vi "LEP_RV_LaunchBuild.vi"(0 "Rebuild":bool, 11 "error in (no error)":errorcluster) -> (4 "Build Result":T1(ring), 15 "error out":errorcluster)   [LabVIEW 2011]
doc: "Loads project configuration information, creates the build folder, prepares the source files, builds, and links the embedded application."
uses:
  <vilib>/LabVIEW Targets/Embedded/ASWServer/MPU_ASWServer_Messages.ctl
  <vilib>/LabVIEW Targets/Embedded/ASWServer/MPU_ASWServer_GeneralIcons.ctl
  <vilib>/LabVIEW Targets/Embedded/ASWServer/MPU_ASWServer_GeneralCtrls.ctl
  LEP_RV_LaunchGlobals.vi
  <vilib>/LabVIEW Targets/Embedded/ASWServer/MPU_ASWServer_General_SetProgressBarValue.vi
  <vilib>/LabVIEW Targets/Embedded/ASWServer/MPU_ASWServer_General_SetProgressBarTitle.vi
panel:
  out "server build output":string
  out "Program Size":string
  out "Build Status":u32(ring)=3 items=["Build OK"=1, "Build OK, with warning(s)"=2, "Build failed with error(s)"=3, "Build cancelled"=4]
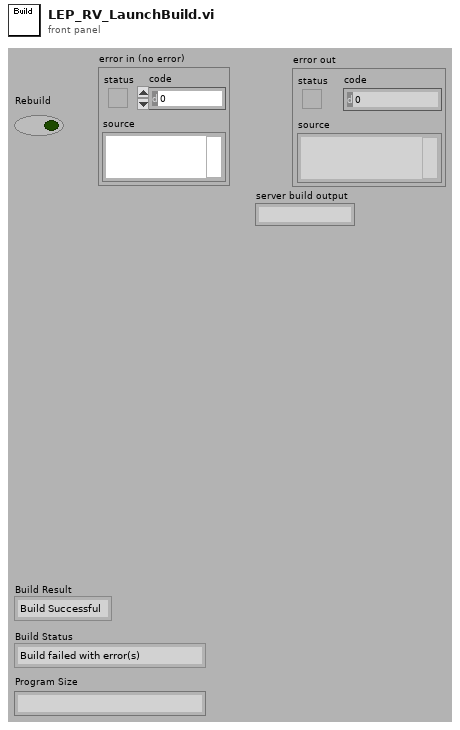
[diagram p1: front panel]
types:
  T1 = enum16{"Build Successful", "Build Failed", "Build Cancelled"}
  T2 = typedef "MPU_ASWServer_Messages.ctl" = enum32{"NoMessage", "Cancel", "ApplicationLaunched"}
  T3 = enum16{"NoErr", "TopLevelVIErr", "EmptyTopLevelVIPath", "CGenErr", "CpySuppFilesErr", "ProjectInfoErr", "NoTopLevelVIErr", "CreateBuildFolderErr", "EmptyBuildFolderErr", "LoadConfigErr", "BildToolsErr", "CompileErr", "LinkError", "DebugInfoErr", "NotFoundErr", "AccessErr", "ExecErr", "UnknownErr", "ISRErr"}
  T4 = enum16{"LoadProjectInfo", "LoadConfig", "SetupBuildFolder", "CopySupportFiles", "CGen", "CreateUVProject", "ConfigureUVproject", "BuildwithUV", "GenerateDebugDatabase", "ShowUserMessage", "Done", "Error"}
  T5 = enum32{"Unused", "OPT_LMISC", "OPT_CMISC", "OPT_AMISC", "OPT_CINCL", "OPT_AINCL", "OPT_CDEF", "OPT_ADEF", "OPT_CUNDEF", "OPT_AUNDEF", "OPT_COPTIMIZE", "OPT_CODEGEN", "OPT_MEMRANGES"}
  T6 = typedef "MPU_ASWServer_GeneralIcons.ctl" = enum16{"Complete", "Disconnected", "Error", "Initializing", "Ready", "Running", "Stopped", "Unknown", "No Change"}
  T7 = typedef "MPU_ASWServer_GeneralCtrls.ctl" = enum16{"Build Status", "Download Status", "Target Name", "Target Type", "Application Name"}
  T8 = enum32{"Unused", "OPT_LMISC", "OPT_CMISC", "OPT_AMISC", "OPT_CINCL", "OPT_AINCL", "OPT_CDEF", "OPT_ADEF", "OPT_CUNDEF", "OPT_AUNDEF", "OPT_COPTIMIZE", "OPT_CODEGEN", "OPT_MEMRANGES", "OPT_ASNMEMRANGES"}
  T9 = typedef "LEP_RV_Config.ctl" = cluster{"Enable debugging":bool, "Debug Options":u16, "Use stack variables":bool, "Generate serial only":bool, "Generate guard code":bool, "Generate Integer Only":bool, "Generate C Function Calls":bool, "ExpressionFolding":bool, "Constant Allocation":u16, "Constant Deallocation":u16, "Build Specification ID":string, "Preprocessor symbols (define)":string, "Compiler Flags":string, "Linker Flags":string, "Mode":u16, "Optimization":u16, "Optimize for time":bool, "Enable cross-module optimization":bool, "Include paths":path[], "Optimize heap size":bool, "Use MicroLib":bool, "Debug Mode":u16, "Enable profile information":bool, "Host name":string, "Use DHCP":bool, "IP address":string, "Subnet mask":string, "Gateway":string, "Primary DNS":string, "Secondary DNS":string, "MAC in target memory":bool, "MAC address":string, "Console output":u16, "Target serial port":u16}
  T10 = cluster{"region name":string, "size":u32, "max":u32, "contains heap?":bool, "RAM?":bool}[]
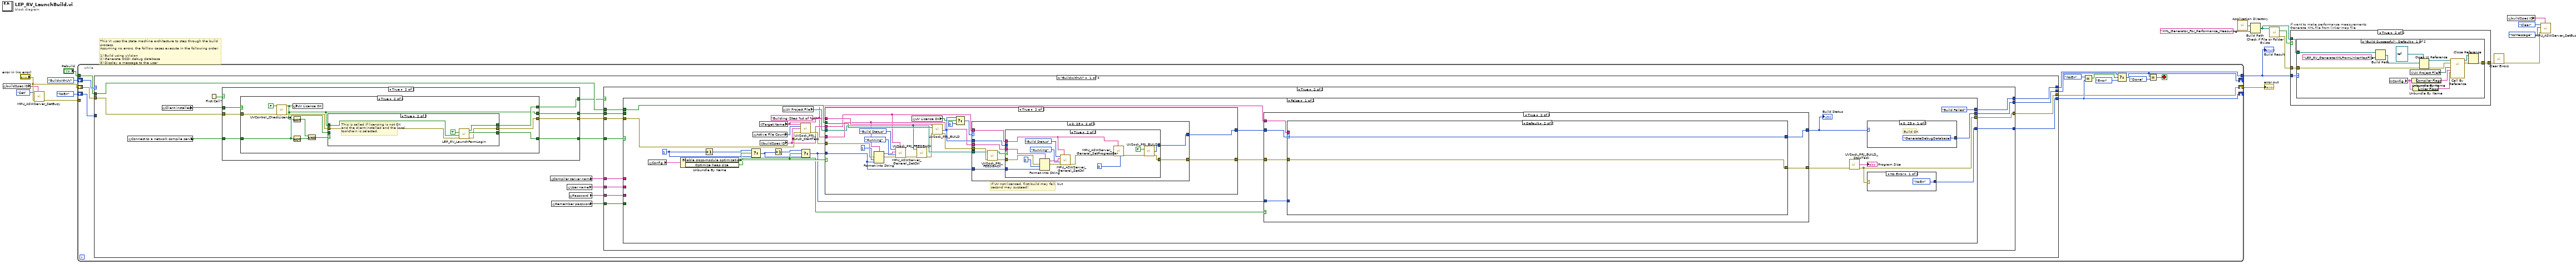
[diagram p0: block diagram]
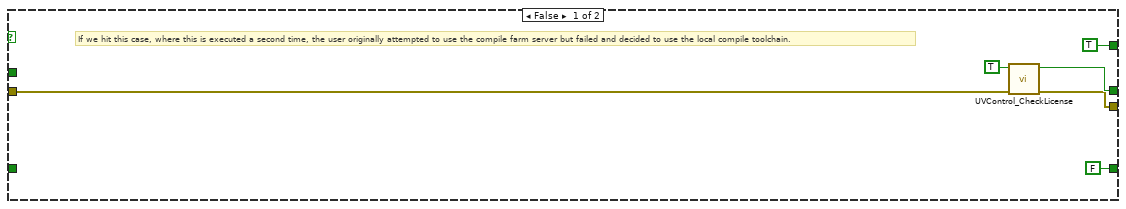
[diagram p4: hidden frame]
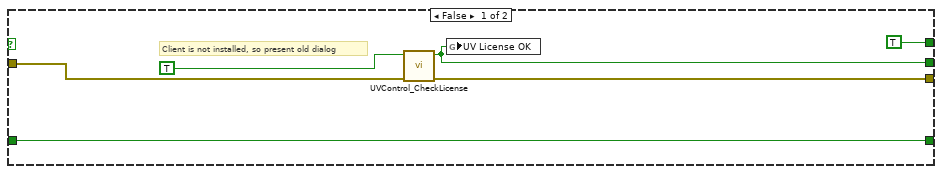
[diagram p5: hidden frame]
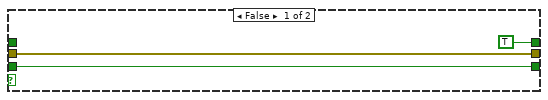
[diagram p6: hidden frame]
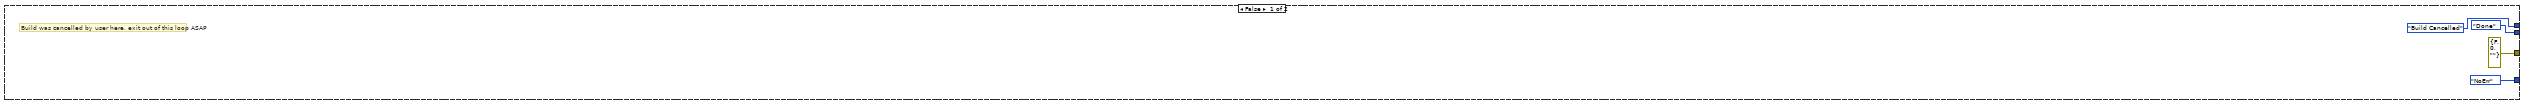
[diagram p7: hidden frame]
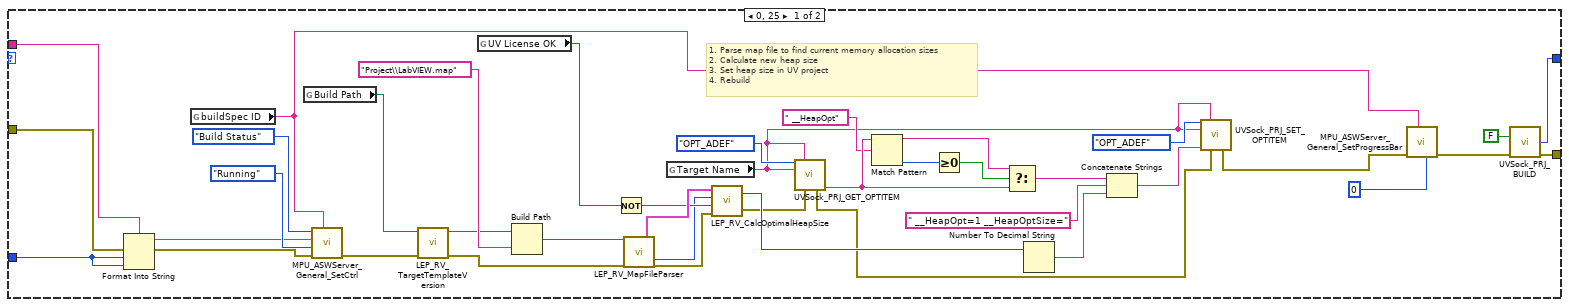
[diagram p9: hidden frame]
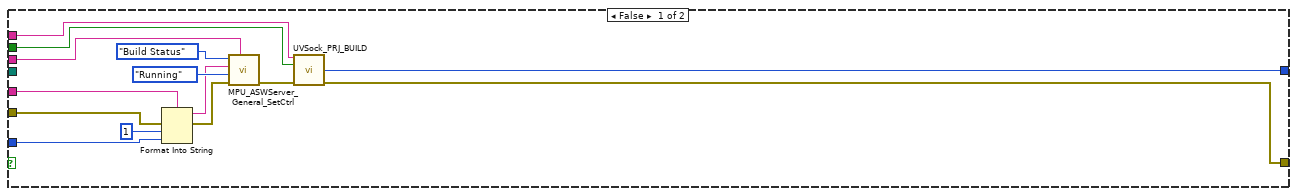
[diagram p10: hidden frame]
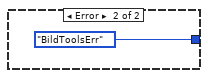
[diagram p13: hidden frame]
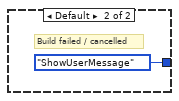
[diagram p14: hidden frame]
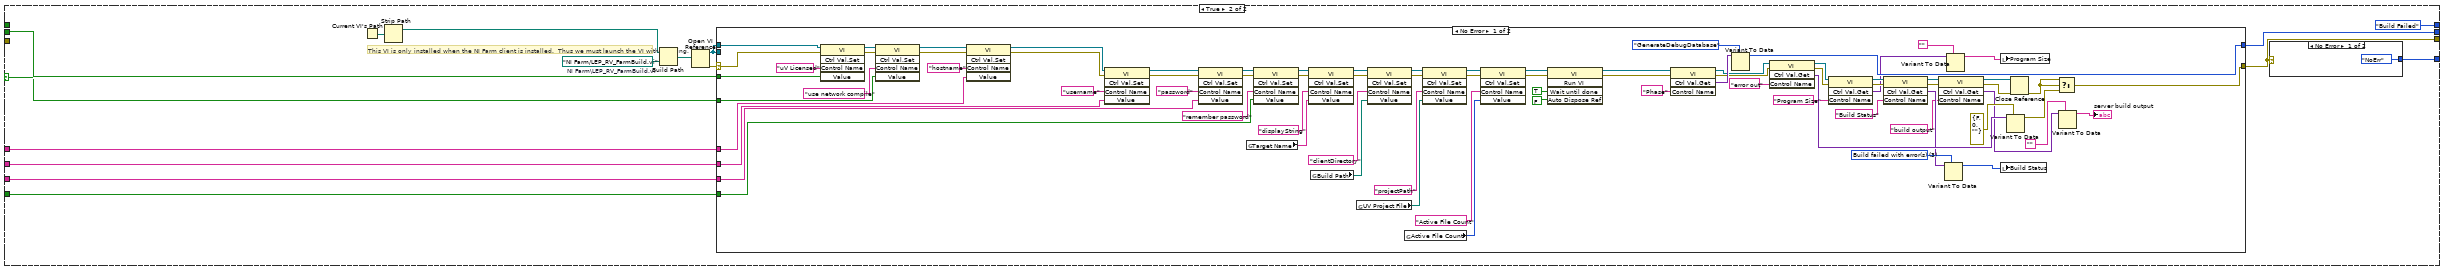
[diagram p15: hidden frame]
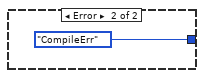
[diagram p16: hidden frame]
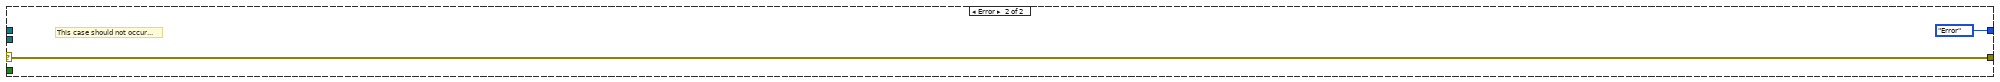
[diagram p17: hidden frame]
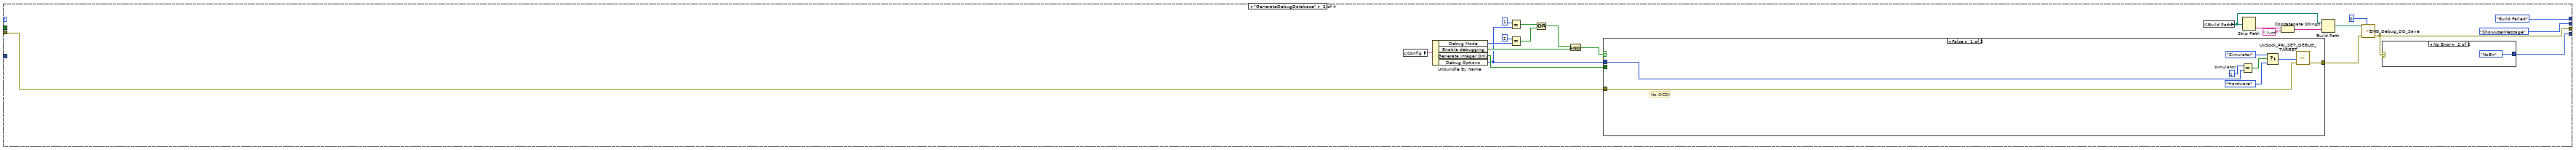
[diagram p18: hidden frame]
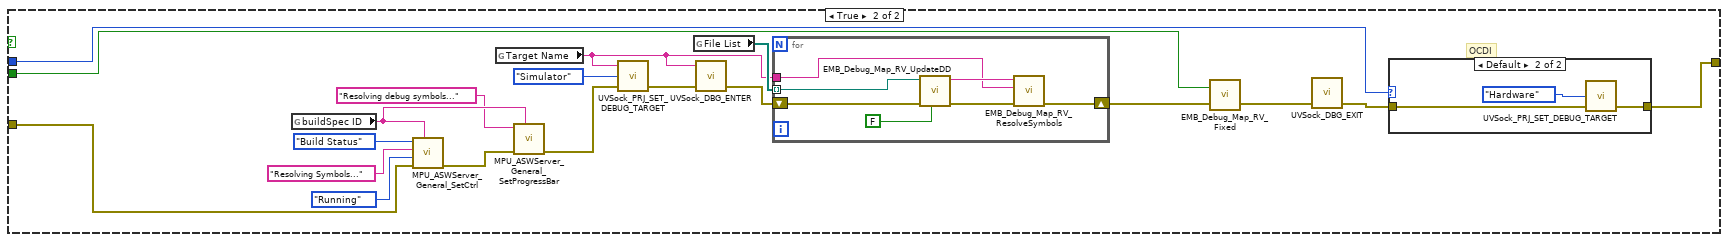
[diagram p19: hidden frame]
diagram:
  # "This VI uses the state machine architecture to step through the build process.\nAssuming no errors, the folllow cases execute in the following order:\n\n1) Build using uVision\n2) Generate OCDI debug database\n3) Display a message to the user"
  n1 = global read "LEP_RV_LaunchGlobals.vi" "buildSpec ID"() -> (w13:string)
  n2 = call <vilib>:"MPU_ASWServer_SetBusy.vi"("buildSpec ID"=w13, "error in (no error)"="error in (no error)", "action"=enum32{"Clear", "Set"}."Set") -> ("error out"=w14:errorcluster)  [unwired: 6 out]
  n3 = while {
    shift-right: [w32] -> w12
    shift-left: "error in (no error)" -> [w20]
    shift-right: [w27] -> _
    shift-left: T4."BuildwithUV" ("Phase") -> [w33]
    shift-right: [w24] -> _
    shift-left: T3."NoErr" ("Errors") -> [w31]
    tunnel: [w25] -> w2
    tunnel: "Rebuild" -> [w22]
    tunnel: w14 -> [_]
    stop <- w28 stop-if-true
    n4 = case shown="\"BuildwithUV\"" w33 {
      tunnel: w20 -> [w45 w358 w414 w539]
      tunnel: [w48 w360 w410 w539] -> w32
      tunnel: [w49 w363 w413 T3."NoErr" ("Errors")] -> w24
      tunnel: w31 -> [_ _ _ w540]
      tunnel: [w46 T4."ShowUserMessage" ("Phase") T4."Done" ("Phase") T4."Done" ("Phase")] -> w29
      tunnel: [w50 T1."Build Failed" ("Build Result") w412 T1."Build Failed" ("Build Result")] -> w25
      tunnel: w22 -> [w47 _ _ _]
      frame "BuildwithUV" {
        n5 = global read "LEP_RV_LaunchGlobals.vi" "Connect to a network compile server"() -> (w41:bool)
        n6 = global read "LEP_RV_LaunchGlobals.vi" "Client installed"() -> (w40:bool)
        n7 = First Call?() -> (First Call?: T/F=w39:bool)
        n8 = case shown="True" w39 {
          tunnel: w45 -> [w54 w63]
          tunnel: [w53 w62] -> w44
          tunnel: [FALSE ("Connect to a network compile server") w61] -> w43
          tunnel: [w55 w60] -> w42
          tunnel: [TRUE ("OK") w59] -> w34
          tunnel: w41 -> [_ w58]
          tunnel: w40 -> [_ w57]
          frame False {
            # "If we hit this case, where this is executed a second time, the user originally attempted to use the compile farm server but failed and decided to use the local compile toolchain."
            n9 = call "UVControl_CheckLicense.vi"("error in (no error)"=w54, "Show Dialog?"=TRUE) -> ("error out"=w53:errorcluster, "License OK"=w55:bool)  [unwired: 8 in]
          }
          frame True {
            n10 = case shown="True" w57 {
              tunnel: w63 -> [w69 w80]
              tunnel: [w68 w78] -> w62
              tunnel: [w65 w70] -> w60
              tunnel: w58 -> [w66 w74]
              tunnel: [w66 w76] -> w61
              tunnel: [TRUE ("OK") w73] -> w59
              frame False {
                # "Client is not installed, so present old dialog"
                n11 = call "UVControl_CheckLicense.vi"("error in (no error)"=w69, "Show Dialog?"=TRUE) -> ("error out"=w68:errorcluster, "License OK"=w65:bool)  [unwired: 8 in]
                n12 = global write "LEP_RV_LaunchGlobals.vi" "UV License OK"(w65) -> ()
              }
              frame True {
                n13 = call "UVControl_CheckLicense.vi"("error in (no error)"=w80, "Show Dialog?"=FALSE) -> ("error out"=w79:errorcluster, "License OK"=w70:bool)  [unwired: 8 in]
                n14 = Not(x=w70) -> (.not. x?=w72:bool)
                n15 = Not(x=w74) -> (.not. x?=w71:bool)
                n16 = global write "LEP_RV_LaunchGlobals.vi" "UV License OK"(w70) -> ()
                n17 = And(x=w72, y=w71) -> (x .and. y?=w75:bool)
                n18 = case shown="True" w75 {
                  tunnel: w79 -> [w83 w86]
                  tunnel: [w83 w87] -> w78
                  tunnel: w74 -> [w82 _]
                  tunnel: [w82 w88] -> w76
                  tunnel: [TRUE ("OK") w89] -> w73
                  tunnel: w70 -> [_ w84]
                  frame False {
                  }
                  frame True {
                    # "This is called if licensing is not OK\nand the client installed and the local\ntoolchain is selected."
                    n19 = call "LEP_RV_LaunchFarmLogin.vi"("error in (no error)"=w86, "uV Licensed"=w84, "build on exit"=TRUE) -> ("error out"=w87:errorcluster, "Connect to a network compile server"=w88:bool, "OK"=w89:bool)  [unwired: 5 in]
                  }
                }
              }
            }
          }
        }
        n20 = global read "LEP_RV_LaunchGlobals.vi" "Compiler server name"() -> (w38:string)
        n21 = global read "LEP_RV_LaunchGlobals.vi" "Remember password"() -> (w35:bool)
        n22 = global read "LEP_RV_LaunchGlobals.vi" "User name"() -> (w37:string)
        n23 = global read "LEP_RV_LaunchGlobals.vi" "Password"() -> (w36:string)
        n24 = case shown="True" w34 {
          tunnel: [T1."Build Cancelled" ("Build Result") w105] -> w50
          tunnel: [T3."NoErr" ("Errors") w104] -> w49
          tunnel: [errorcluster {"status"=FALSE, "code"=0, "source"=""} ("error IO") w103] -> w48
          tunnel: w47 -> [_ w102]
          tunnel: [T4."Done" ("Phase") w101] -> w46
          tunnel: w44 -> [_ w100]
          tunnel: w43 -> [_ w99]
          tunnel: w42 -> [_ w98]
          tunnel: w38 -> [_ w97]
          tunnel: w37 -> [_ w96]
          tunnel: w36 -> [_ w95]
          tunnel: w35 -> [_ w94]
          frame False {
            # "Build was cancelled by user here, exit out of this loop ASAP"
          }
          frame True {
            n25 = case shown="False" w99 {
              selector: w99 -> [_ w254]
              tunnel: [T1."Build Failed" ("Build Result") T1."Build Failed" ("Build Result")] -> w105
              tunnel: [w129 w259] -> w104
              tunnel: [w128 w257] -> w103
              tunnel: w102 -> [w127 _]
              tunnel: [w125 w256] -> w101
              tunnel: w100 -> [w106 _]
              tunnel: w98 -> [_ w255]
              tunnel: w97 -> [_ w253]
              tunnel: w96 -> [_ w252]
              tunnel: w95 -> [_ w251]
              tunnel: w94 -> [_ w250]
              frame False {
                w107 = "Building (Step %d of %d)" ("format string")
                w112 = 1
                n26 = global read "LEP_RV_LaunchGlobals.vi" "Config"() -> (w119:T9)
                n27 = Unbundle By Name(w119) -> ("Enable cross-module optimization"=w114:bool, "Optimize heap size"=w110:bool)
                n28 = Increment(x=w112) -> (x+1=w113:i32)
                n29 = Select(t=w113, s=w114, f=w112) -> (s? t:f=w109:i32)
                n30 = global read "LEP_RV_LaunchGlobals.vi" "Active File Count"() -> (w120:i32)
                n31 = global read "LEP_RV_LaunchGlobals.vi" "Target Name"() -> (w122:string)
                n32 = global read "LEP_RV_LaunchGlobals.vi" "buildSpec ID"() -> (w121:string)
                n33 = Increment(x=w109) -> (x+1=w111:i32)
                n34 = global read "LEP_RV_LaunchGlobals.vi" "UV Project File"() -> (w123:path)
                n35 = call "UVSock_PRJ_BUILD_StartTask.vi"("Target"=w122, "Active File Count"=w120, "buildSpec ID"=w121, "error in (no error)"=w106) -> ("error out"=w124:errorcluster)  [unwired: 11 out]
                n36 = Select(t=w111, s=w110, f=w109) -> (s? t:f=w108:i32)
                n37 = case shown="True" w114 {
                  tunnel: w127 -> [w193 w215]
                  tunnel: w124 -> [w183 w198]
                  tunnel: w123 -> [_ w214]
                  tunnel: [w192 w213] -> w116
                  tunnel: w122 -> [w194 w200]
                  tunnel: [w191 w212] -> w118
                  tunnel: w121 -> [w185 w195]
                  tunnel: w108 -> [w184 w196]
                  tunnel: w107 -> [w182 w197]
                  frame False {
                    n38 = Format Into String(format string=w182, error in=w183, 1, w184) -> (resulting string=w186:string, error out=w187:errorcluster)  [unwired: 1 in]
                    n39 = call <vilib>:"MPU_ASWServer_General_SetCtrl.vi"("buildSpec ID"=w185, "error in"=w187, "icon"=MPU_ASWServer_GeneralIcons."Running" ("Icon"), "value"=w186, "control"=MPU_ASWServer_GeneralCtrls."Build Status" ("Control")) -> ("error out"=w181:errorcluster)  [unwired: 4 in, 2 out]
                    n40 = call "UVSock_PRJ_BUILD.vi"("Target"=w194, "Rebuild"=w193, "error in (no error)"=w181) -> ("Build Status"=w191:u32, "error out"=w192:errorcluster)  [unwired: 11 out]
                  }
                  frame True {
                    # "If UV not licensed, first build may fail, but\nsecond may succeed!"
                    n41 = Format Into String(format string=w197, error in=w198, 1, w196) -> (resulting string=w199:string, error out=w201:errorcluster)  [unwired: 1 in]
                    n42 = call <vilib>:"MPU_ASWServer_General_SetCtrl.vi"("buildSpec ID"=w195, "error in"=w201, "icon"=MPU_ASWServer_GeneralIcons."Running" ("Icon"), "value"=w199, "control"=MPU_ASWServer_GeneralCtrls."Build Status" ("Control")) -> ("error out"=w203:errorcluster)  [unwired: 4 in, 2 out]
                    n43 = global read "LEP_RV_LaunchGlobals.vi" "UV License OK"() -> (w206:bool)
                    n44 = call "UVSock_PRJ_FEEDBACK.vi"("error in (no error)"=w203, "Path"=w214) -> ("error out"=w211:errorcluster)  [unwired: 9 out]
                    n45 = call "UVSock_PRJ_BUILD.vi"("Target"=w200, "Rebuild"=w215, "error in (no error)"=w211) -> ("Build Status"=w207:u32, "error out"=w210:errorcluster)  [unwired: 11 out]
                    n46 = Select(t=w207, s=w206, f=u32 0) -> (s? t:f=w209:u32)
                    n47 = case shown="0, 25" w209 {
                      selector: w209 -> [w217 _]
                      tunnel: w210 -> [w216 w227]
                      tunnel: w214 -> [_ w226]
                      tunnel: [w216 w224] -> w213
                      tunnel: [w217 w222] -> w212
                      tunnel: w207 -> [_ w221]
                      tunnel: w195 -> [_ w220]
                      tunnel: w197 -> [_ w219]
                      tunnel: w196 -> [_ w218]
                      frame Default {
                      }
                      frame 0, 25 {
                        n48 = call "UVSock_PRJ_FEEDBACK.vi"("error in (no error)"=w227, "Path"=w226) -> ("error out"=w225:errorcluster, "new feedback data?"=w223:bool)  [unwired: 8 out]
                        n49 = case shown="True" w223 {
                          tunnel: w225 -> [w229 w234]
                          tunnel: [w229 w244] -> w224
                          tunnel: [w228 w243] -> w222
                          tunnel: w221 -> [w228 _]
                          tunnel: w220 -> [_ w232]
                          tunnel: w219 -> [_ w231]
                          tunnel: w218 -> [_ w235]
                          frame False {
                          }
                          frame True {
                            n50 = Format Into String(format string=w231, error in=w234, 2, w235) -> (resulting string=w240:string, error out=w239:errorcluster)  [unwired: 1 in]
                            n51 = call <vilib>:"MPU_ASWServer_General_SetCtrl.vi"("buildSpec ID"=w232, "error in"=w239, "icon"=MPU_ASWServer_GeneralIcons."Running" ("Icon"), "value"=w240, "control"=MPU_ASWServer_GeneralCtrls."Build Status" ("Control")) -> ("error out"=w233:errorcluster)  [unwired: 4 in, 2 out]
                            n52 = call-poly <vilib>:"MPU_ASWServer_General_SetProgressBar.vi"("value"=u32 0, "buildSpec ID"=w232, "error in"=w233) -> ("error out"=w242:errorcluster)  [unwired: 6 in, 2 out]
                            n53 = call "UVSock_PRJ_BUILD.vi"("Rebuild"=FALSE, "error in (no error)"=w242) -> ("Build Status"=w243:u32, "error out"=w244:errorcluster)  [unwired: 1 in, 11 out]
                          }
                        }
                      }
                    }
                  }
                }
                n54 = case shown="True" w110 {
                  tunnel: w118 -> [w132 w138]
                  tunnel: w116 -> [w131 w136]
                  tunnel: [w132 w137] -> w117
                  tunnel: [w131 w135] -> w115
                  tunnel: w108 -> [_ w134]
                  tunnel: w107 -> [_ w133]
                  frame False {
                  }
                  frame True {
                    n55 = case shown="Default" w138 {
                      selector: w138 -> [_ w180]
                      tunnel: [w172 w180] -> w137
                      tunnel: w136 -> [w153 w179]
                      tunnel: [w173 w179] -> w135
                      tunnel: w134 -> [w152 _]
                      tunnel: w133 -> [w151 _]
                      frame 0, 25 {
                        # "1. Parse map file to find current memory allocation sizes\n2. Calculate new heap size\n3. Set heap size in UV project\n4. Rebuild"
                        n56 = Format Into String(format string=w151, error in=w153, w152, w152) -> (resulting string=w156:string, error out=w157:errorcluster)  [unwired: 1 in]
                        n57 = global read "LEP_RV_LaunchGlobals.vi" "buildSpec ID"() -> (w155:string)
                        n58 = global read "LEP_RV_LaunchGlobals.vi" "Build Path"() -> (w178:path)
                        n59 = call <vilib>:"MPU_ASWServer_General_SetCtrl.vi"("buildSpec ID"=w155, "error in"=w157, "icon"=MPU_ASWServer_GeneralIcons."Running" ("Icon"), "value"=w156, "control"=MPU_ASWServer_GeneralCtrls."Build Status" ("Control")) -> ("error out"=w154:errorcluster)  [unwired: 4 in, 2 out]
                        n60 = call "LEP_RV_TargetTemplateVersion.vi"("error in (no error)"=w154, "Path"=w178) -> ("error out"=w175:errorcluster, "Path plus Version"=w176:path)  [unwired: 7 in, 1 out]
                        n61 = global read "LEP_RV_LaunchGlobals.vi" "UV License OK"() -> (w162:bool)
                        n62 = Build Path(base path=w176, name or relative path="Project\\LabVIEW.map") -> (appended path=w174:path)
                        n63 = Not(x=w162) -> (.not. x?=w161:bool)
                        n64 = call "LEP_RV_MapFileParser.vi"("map file"=w174, "error in (no error)"=w175) -> ("regions"=w164:T10, "heap size"=w160:i32, "error out"=w163:errorcluster)  [unwired: 11 in, 4 out]
                        n65 = global read "LEP_RV_LaunchGlobals.vi" "Target Name"() -> (w141:string)
                        n66 = call "LEP_RV_CalcOptimalHeapSize.vi"("error in (no error)"=w163, "eval mode?"=w161, "heap size"=w160, "memory regions"=w164) -> ("error out"=w140:errorcluster, "optimal heap size"=w165:u32)
                        n67 = call "UVSock_PRJ_GET_OPTITEM.vi"("Option In"=T5."OPT_ADEF", "Target"=w141, "Target Name In"=w141, "error in (no error)"=w140) -> ("error out"=w139:errorcluster, "Item Out"=w148:string)  [unwired: 9 in, 1 out]
                        n68 = Match Pattern(string=w148, regular expression=" __HeapOpt") -> (before substring=w149:string, offset past match=w147:i32)  [unwired: 1 in, 2 out]
                        n69 = Greater Or Equal To 0?(x=w147) -> (x >= 0?=w146:bool)
                        n70 = Select(t=w149, s=w146, f=w148) -> (s? t:f=w143:string)
                        n71 = Number To Decimal String(number=w165) -> (decimal integer string=w167:string)  [unwired: 1 in]
                        n72 = Concatenate Strings(w143, " __HeapOpt=1 __HeapOptSize=" ("string"), w167) -> (w142:string)
                        n73 = call "UVSock_PRJ_SET_OPTITEM.vi"("Option In"=T8."OPT_ADEF", "Target"=w141, "Target Name In"=w141, "Item In"=w142, "error in (no error)"=w139) -> ("error out"=w168:errorcluster)  [unwired: 10 in]
                        n74 = call-poly <vilib>:"MPU_ASWServer_General_SetProgressBar.vi"("value"=u32 0, "buildSpec ID"=w155, "error in"=w168) -> ("error out"=w170:errorcluster)  [unwired: 6 in, 2 out]
                        n75 = call "UVSock_PRJ_BUILD.vi"("Rebuild"=FALSE, "error in (no error)"=w170) -> ("Build Status"=w172:u32, "error out"=w173:errorcluster)  [unwired: 1 in, 11 out]
                      }
                      frame Default {
                      }
                    }
                  }
                }
                "Build Status" <- w117
                n76 = call "UVSock_PRJ_BUILD_StopTask.vi"("error in (no error)"=w115) -> ("error out"=w128:errorcluster, "Program Size"=→"Program Size":string)  [unwired: 3 out]
                n77 = case shown="0, 25" w117 {
                  tunnel: [T4."GenerateDebugDatabase" ("Phase") T4."ShowUserMessage" ("Phase")] -> w125
                  frame 0, 25 {
                    # "Build OK"
                  }
                  frame Default {
                    # "Build failed / cancelled"
                  }
                }
                n78 = case shown="No Error" w128 {
                  tunnel: [T3."NoErr" ("Errors") T3."BildToolsErr" ("Errors")] -> w129
                  frame No Error {
                  }
                  frame Error {
                  }
                }
              }
              frame True {
                w264 = path "NI Farm/LEP_RV_FarmBuild.vi"  # NI Farm\LEP_RV_FarmBuild.vi
                # "This VI is only installed when the NI Farm client is installed.  Thus we must launch the VI with scripting."
                n79 = Current VI's Path() -> (path=w263:path)
                n80 = Strip Path(path=w263) -> (stripped path=w262:path)  [unwired: 1 out]
                n81 = Build Path(base path=w262, name or relative path=w264) -> (appended path=w261:path)
                n82 = Open VI Reference(vi path=w261) -> (vi reference=w249:refnum<vi>, error out=w260:errorcluster)  [unwired: 5 in]
                n83 = case shown="No Error" w260 {
                  selector: w260 -> [w338 w346]
                  tunnel: w249 -> [w339 _]
                  tunnel: [w325 w346] -> w257
                  tunnel: [w333 T4."Error" ("Phase")] -> w256
                  tunnel: w255 -> [w337 _]
                  tunnel: w254 -> [w303 _]
                  tunnel: w253 -> [w302 _]
                  tunnel: w252 -> [w301 _]
                  tunnel: w251 -> [w300 _]
                  tunnel: w250 -> [w299 _]
                  tunnel: w249 -> [_ _]
                  frame No Error {
                    w283 = u32 3 items=["Build OK"=1, "Build OK, with warning(s)"=2, "Build failed with error(s)"=3, "Build cancelled"=4] ("Build Status")
                    n84 = invoke class="VI" method="Ctrl Val.Set"(reference=w339, error in=w338, "Control Name"="uV Licensed", "Value"=w337) -> (reference out=w305:refnum<vi>, error out=w304:errorcluster)  [unwired: 1 in, 3 out]
                    n85 = invoke class="VI" method="Ctrl Val.Set"(reference=w305, error in=w304, "Control Name"="use network compile", "Value"=w303) -> (reference out=w309:refnum<vi>, error out=w308:errorcluster)  [unwired: 1 in, 3 out]
                    n86 = invoke class="VI" method="Ctrl Val.Set"(reference=w309, error in=w308, "Control Name"="hostname", "Value"=w302) -> (reference out=w311:refnum<vi>, error out=w310:errorcluster)  [unwired: 1 in, 3 out]
                    n87 = invoke class="VI" method="Ctrl Val.Set"(reference=w311, error in=w310, "Control Name"="username", "Value"=w301) -> (reference out=w313:refnum<vi>, error out=w312:errorcluster)  [unwired: 1 in, 3 out]
                    n88 = invoke class="VI" method="Ctrl Val.Set"(reference=w313, error in=w312, "Control Name"="password", "Value"=w300) -> (reference out=w315:refnum<vi>, error out=w314:errorcluster)  [unwired: 1 in, 3 out]
                    n89 = global read "LEP_RV_LaunchGlobals.vi" "Target Name"() -> (w297:string)
                    n90 = invoke class="VI" method="Ctrl Val.Set"(reference=w315, error in=w314, "Control Name"="remember password", "Value"=w299) -> (reference out=w317:refnum<vi>, error out=w316:errorcluster)  [unwired: 1 in, 3 out]
                    n91 = invoke class="VI" method="Ctrl Val.Set"(reference=w317, error in=w316, "Control Name"="displayString", "Value"=w297) -> (reference out=w307:refnum<vi>, error out=w306:errorcluster)  [unwired: 1 in, 3 out]
                    n92 = global read "LEP_RV_LaunchGlobals.vi" "Build Path"() -> (w298:path)
                    n93 = global read "LEP_RV_LaunchGlobals.vi" "UV Project File"() -> (w293:path)
                    n94 = invoke class="VI" method="Ctrl Val.Set"(reference=w307, error in=w306, "Control Name"="clientDirectory", "Value"=w298) -> (reference out=w296:refnum<vi>, error out=w295:errorcluster)  [unwired: 1 in, 3 out]
                    n95 = global read "LEP_RV_LaunchGlobals.vi" "Active File Count"() -> (w275:i32)
                    n96 = invoke class="VI" method="Ctrl Val.Set"(reference=w296, error in=w295, "Control Name"="projectPath", "Value"=w293) -> (reference out=w280:refnum<vi>, error out=w279:errorcluster)  [unwired: 1 in, 3 out]
                    n97 = invoke class="VI" method="Ctrl Val.Set"(reference=w280, error in=w279, "Control Name"="Active File Count", "Value"=w275) -> (reference out=w278:refnum<vi>, error out=w277:errorcluster)  [unwired: 1 in, 3 out]
                    n98 = invoke class="VI" method="Run VI"(reference=w278, error in=w277, "Wait until done"=TRUE ("Wait Until Done"), "Auto Dispose Ref"=FALSE ("Auto Dispose Reference")) -> (reference out=w342:refnum<vi>, error out=w341:errorcluster)  [unwired: 1 in, 3 out]
                    n99 = invoke class="VI" method="Ctrl Val.Get"(reference=w342, error in=w341, "Control Name"="Phase") -> (reference out=w332:refnum<vi>, error out=w331:errorcluster, "Get Control Value Variant"=w334:variant)  [unwired: 1 in, 1 out]
                    n100 = Variant To Data(type=T4."GenerateDebugDatabase" ("Phase"), Variant=w334) -> (data=w333:T4)  [unwired: 1 in, 1 out]
                    n101 = invoke class="VI" method="Ctrl Val.Get"(reference=w332, error in=w331, "Control Name"="error out") -> (reference out=w292:refnum<vi>, error out=w290:errorcluster, "Get Control Value Variant"=w328:variant)  [unwired: 1 in, 1 out]
                    n102 = invoke class="VI" method="Ctrl Val.Get"(reference=w292, error in=w290, "Control Name"="Program Size") -> (reference out=w291:refnum<vi>, error out=w289:errorcluster, "Get Control Value Variant"=w285:variant)  [unwired: 1 in, 1 out]
                    n103 = invoke class="VI" method="Ctrl Val.Get"(reference=w291, error in=w289, "Control Name"="Build Status") -> (reference out=w274:refnum<vi>, error out=w273:errorcluster, "Get Control Value Variant"=w282:variant)  [unwired: 1 in, 1 out]
                    n104 = invoke class="VI" method="Ctrl Val.Get"(reference=w274, error in=w273, "Control Name"="build output") -> (reference out=w272:refnum<vi>, error out=w271:errorcluster, "Get Control Value Variant"=w269:variant)  [unwired: 1 in, 1 out]
                    n105 = Variant To Data(type=w283, Variant=w282) -> (data=w281:u32)  [unwired: 1 in, 1 out]
                    n106 = Variant To Data(type="" ("Program Size"), Variant=w285) -> (data=w284:string)  [unwired: 1 in, 1 out]
                    n107 = local write "Program Size"(w284) -> ()
                    n108 = local write "Build Status"(w281) -> ()
                    n109 = Variant To Data(type=errorcluster {"status"=FALSE, "code"=0, "source"=""} ("error out"), Variant=w328) -> (data=w326:errorcluster)  [unwired: 1 in, 1 out]
                    n110 = Close Reference(reference=w272, error in (no error)=w271) -> (error out=w327:errorcluster)
                    n111 = Select(t=w327, s=w327, f=w326) -> (s? t:f=w325:errorcluster)
                    n112 = Variant To Data(type="", Variant=w269) -> (data=→"server build output":string)  [unwired: 1 in, 1 out]
                  }
                  frame Error {
                    # "This case should not occur..."
                  }
                }
                n113 = case shown="No Error" w257 {
                  tunnel: [T3."NoErr" ("Errors") T3."CompileErr" ("Errors")] -> w259
                  frame No Error {
                  }
                  frame Error {
                  }
                }
              }
            }
          }
        }
      }
      frame "GenerateDebugDatabase" {
        n114 = global read "LEP_RV_LaunchGlobals.vi" "Config"() -> (w348:T9)
        n115 = Unbundle By Name(w348) -> ("Debug Mode"=w354:u16, "Enable debugging"=w356:bool, "Generate Integer Only"=w359:bool, "Debug Options"=w349:u16)
        n116 = Equal?(x=u16 1, y=w349) -> (x = y?=w351:bool)
        n117 = Equal?(x=u16 2, y=w354) -> (x = y?=w355:bool)
        n118 = Or(x=w351, y=w355) -> (x .or. y?=w352:bool)
        n119 = And(x=w352, y=w356) -> (x .and. y?=w357:bool)
        n120 = case shown="False" w357 {
          tunnel: w358 -> [w377 w386]
          tunnel: [w376 w385] -> w361
          tunnel: w359 -> [_ w395]
          tunnel: w349 -> [w371 w391]
          frame False {
            w370 = u16 1  # simulator
            # "No OCDI"
            n121 = Equal?(x=w370, y=w371) -> (x = y?=w372:bool)
            n122 = Select(t=enum16{"Hardware", "Simulator"}."Simulator" ("Debug Target"), s=w372, f=enum16{"Hardware", "Simulator"}."Hardware") -> (s? t:f=w374:enum16{"Hardware", "Simulator"})
            n123 = call "UVSock_PRJ_SET_DEBUG_TARGET.vi"("error in (no error)"=w377, "Debug Target"=w374) -> ("error out"=w376:errorcluster)  [unwired: 1 in, 2 out]
          }
          frame True {
            # "OCDI"
            n124 = global read "LEP_RV_LaunchGlobals.vi" "buildSpec ID"() -> (w379:string)
            n125 = call <vilib>:"MPU_ASWServer_General_SetCtrl.vi"("buildSpec ID"=w379, "error in"=w386, "icon"=MPU_ASWServer_GeneralIcons."Running" ("Icon"), "value"="Resolving Symbols...", "control"=MPU_ASWServer_GeneralCtrls."Build Status" ("Control")) -> ("error out"=w381:errorcluster)  [unwired: 4 in, 2 out]
            n126 = global read "LEP_RV_LaunchGlobals.vi" "Target Name"() -> (w382:string)
            n127 = call-poly <vilib>:"MPU_ASWServer_General_SetProgressBar.vi"("buildSpec ID"=w379, "error in"=w381, "title"="Resolving debug symbols...") -> ("error out"=w380:errorcluster)  [unwired: 6 in, 2 out]
            n128 = call "UVSock_PRJ_SET_DEBUG_TARGET.vi"("error in (no error)"=w380, "Debug Target"=enum16{"Hardware", "Simulator"}."Simulator", "Target"=w382) -> ("error out"=w393:errorcluster)  [unwired: 2 out]
            n129 = global read "LEP_RV_LaunchGlobals.vi" "File List"() -> (w383:path[])
            n130 = call "UVSock_DBG_ENTER.vi"("error in (no error)"=w393, "Target"=w382) -> ("error out"=w384:errorcluster)  [unwired: 3 out]
            n131 = for {
              tunnel: w383 -> [w404] mode=indexing
              shift-right: [w402] -> w396
              shift-left: w384 -> [w407]
              tunnel: w382 -> [w401]
              n132 = call "EMB_Debug_Map_RV_UpdateDD.vi"("RDM"=FALSE, "error in (no error)"=w407, "Source Path"=w404) -> ("error out"=w405:errorcluster, "VI Name"=w403:string)  [unwired: 2 in, 5 out]
              n133 = call "EMB_Debug_Map_RV_ResolveSymbols.vi"("error in (no error)"=w405, "Target"=w401, "VI Name"=w403) -> ("error out"=w402:errorcluster)  [unwired: 8 out]
            }
            n134 = call "EMB_Debug_Map_RV_Fixed.vi"("error in (no error)"=w396, "Generate Integer Only"=w395) -> ("error out"=w394:errorcluster)  [unwired: 1 out]
            n135 = call "UVSock_DBG_EXIT.vi"("error in (no error)"=w394) -> ("error out"=w390:errorcluster)  [unwired: 1 in, 3 out]
            n136 = case shown="Default" w391 {
              tunnel: w390 -> [w397 w399]
              tunnel: [w397 w398] -> w385
              frame 1 {
              }
              frame Default {
                n137 = call "UVSock_PRJ_SET_DEBUG_TARGET.vi"("error in (no error)"=w399, "Debug Target"=enum16{"Hardware", "Simulator"}."Hardware") -> ("error out"=w398:errorcluster)  [unwired: 1 in, 2 out]
              }
            }
          }
        }
        n138 = global read "LEP_RV_LaunchGlobals.vi" "Build Path"() -> (w347:path)
        n139 = Strip Path(path=w347) -> (name=w366:string)  [unwired: 1 out]
        n140 = Concatenate Strings(w366, ".lvm" ("name or relative path")) -> (w368:string)
        n141 = Build Path(base path=w347, name or relative path=w368) -> (appended path=w365:path)
        n142 = call <vilib>:"EMB_Debug_DD_Save.vi"("target ID"=u32 0, "error in (no error)"=w361, "Path"=w365) -> ("error out"=w360:errorcluster)  [unwired: 8 out]
        n143 = case shown="No Error" w360 {
          tunnel: [T3."NoErr" ("Errors") T3."DebugInfoErr" ("Errors")] -> w363
          frame No Error {
          }
          frame Error {
          }
        }
      }
      frame "ShowUserMessage" {
        n144 = case "Show the correct dialogs for the build result" shown="No Error" w414 {
          tunnel: [T3."NoErr" ("Errors") T3."BildToolsErr" ("Errors")] -> w413
          tunnel: [w422 T1."Build Failed" ("Build Result")] -> w412
          tunnel: [w418 _] -> w410
          frame No Error {
            n145 = global read "LEP_RV_LaunchGlobals.vi" "buildSpec ID"() -> (w415:string)
            n146 = local read "Program Size"() -> (w420:string)
            n147 = local read "Build Status"() -> (w421:u32)
            n148 = call-poly <vilib>:"MPU_ASWServer_General_SetProgressBar.vi"("value"=u32 0, "buildSpec ID"=w415) -> ("error out"=w417:errorcluster)  [unwired: 7 in, 2 out]
            n149 = case shown="26, Default" w421 {
              tunnel: [T1."Build Successful" ("Build Result") T1."Build Failed" ("Build Result") T1."Build Cancelled" ("Build Result")] -> w422
              tunnel: w420 -> [_ _ _]
              tunnel: w415 -> [w426 w461 w500]
              tunnel: [w439 errorcluster {"status"=TRUE, "code"=42, "source"="failed"} ("error out") errorcluster {"status"=TRUE, "code"=42, "source"="Cancelled"} ("error out")] -> w418
              tunnel: w417 -> [w442 w484 w507]
              frame 0, 25 {
                w427 = "Build Report" ("tab name")
                w449 = "Output" ("tab name")
                n150 = Get Date/Time In Seconds() -> (seconds since 1Jan1904=w444:timestamp)
                n151 = Get Date/Time String(seconds (now)=w444, want seconds? (F)=TRUE) -> (time string=w448:string)  [unwired: 2 out]
                n152 = Concatenate Strings("[" ("string"), w448, "]" ("string"), " Status: Build Succeeded." ("string"), "\r\n") -> (w452:string)
                n153 = call <vilib>:"MPU_ASWServer_Send.vi"("generate events? (F)"=TRUE ("show tab? (F)"), "wait for ACK (T)"=FALSE, "buildSpec ID"=w426, "error in"=w442, "control value"=w452, "control name"=w449, "tab name"=w449) -> ("error out"=w441:errorcluster)  [unwired: 4 out]
                n154 = global read "LEP_RV_LaunchGlobals.vi" "UV License OK"() -> (w429:bool)
                n155 = call-poly <vilib>:"MPU_ASWServer_General_SetProgressBar.vi"("buildSpec ID"=w426, "error in"=w441, "title"="Done") -> ("error out"=w453:errorcluster)  [unwired: 6 in, 2 out]
                n156 = call <vilib>:"MPU_ASWServer_General_SetCtrl.vi"("buildSpec ID"=w426, "error in"=w453, "icon"=MPU_ASWServer_GeneralIcons."Running" ("Icon"), "value"="Build Succeeded" ("Value"), "control"=MPU_ASWServer_GeneralCtrls."Build Status" ("Control")) -> ("error out"=w431:errorcluster)  [unwired: 4 in, 2 out]
                n157 = Not(x=w429) -> (.not. x?=w428:bool)
                n158 = global read "LEP_RV_LaunchGlobals.vi" "Build Path"() -> (w433:path)
                n159 = call "LEP_RV_TargetTemplateVersion.vi"("Path"=w433) -> ("Path plus Version"=w432:path)  [unwired: 8 in, 2 out]
                n160 = call <vilib>:"MPU_ASWServer_Send.vi"("generate events? (F)"=FALSE, "wait for ACK (T)"=FALSE, "buildSpec ID"=w426, "error in"=w431, "control value"=w428, "control name"="eval mode?", "tab name"=w427) -> ("error out"=w430:errorcluster)  [unwired: 4 out]
                n161 = Build Path(base path=w432, name or relative path="Project\\LabVIEW.map") -> (appended path=w434:path)
                n162 = call <vilib>:"MPU_ASWServer_Send.vi"("generate events? (F)"=TRUE, "wait for ACK (T)"=FALSE, "buildSpec ID"=w426, "error in"=w430, "control value"=w434, "control name"="path to map file", "tab name"=w427) -> ("error out"=w439:errorcluster)  [unwired: 4 out]
              }
              frame 26, Default {
                w482 = "\r\n"
                n163 = global read "LEP_RV_LaunchGlobals.vi" "Connect to a network compile server"() -> (w459:bool)
                n164 = case shown="False" w459 {
                  tunnel: [w493 w494] -> w478
                  frame False {
                    n165 = call "UVSock_GetBuildOutput.vi"() -> ("Build Output"=w493:string)  [unwired: 2 in, 3 out]
                  }
                  frame True {
                    n166 = local read "server build output"() -> (w494:string)
                  }
                }
                n167 = Match Pattern(string=w478, regular expression="linking...") -> (before substring=w473:string, match substring=w475:string, after substring=w474:string, offset past match=w476:i32)  [unwired: 1 in]
                n168 = case shown="Default" w476 {
                  tunnel: w475 -> [w497 _]
                  tunnel: w474 -> [w496 _]
                  tunnel: w473 -> [_ w498]
                  tunnel: [w495 w498] -> w469
                  frame Default {
                    n169 = Concatenate Strings(w497, w496) -> (w495:string)
                  }
                  frame -1 {
                  }
                }
                n170 = Match Pattern(string=w469, regular expression="L6406W") -> (offset past match=w471:i32)  [unwired: 1 in, 3 out]
                n171 = Greater Or Equal To 0?(x=w471) -> (x >= 0?=w470:bool)
                n172 = Select(t="linking...\nError: Application is too large for target memory.", s=w470, f=w469) -> (s? t:f=w467:string)
                n173 = Concatenate Strings(w467, w482, "Status: Build failed." ("string"), w482) -> (w481:string)
                n174 = call <vilib>:"MPU_ASWServer_General_SetCtrl.vi"("buildSpec ID"=w461, "error in"=w484, "icon"=MPU_ASWServer_GeneralIcons."Error", "value"="Build Failed", "control"=MPU_ASWServer_GeneralCtrls."Build Status") -> ("error out"=w488:errorcluster)  [unwired: 4 in, 2 out]
                n175 = String Subset(string=w481, length (rest)=30000 ("length (rest)")) -> (substring=w480:string)  [unwired: 1 in]
                n176 = call-poly <vilib>:"MPU_ASWServer_General_SetProgressBar.vi"("buildSpec ID"=w461, "error in"=w488, "title"="Failed") -> ("error out"=w489:errorcluster)  [unwired: 6 in, 2 out]
                n177 = call <vilib>:"MPU_ASWServer_Output_SetError.vi"("error in"=w489, "error str"=w480, "buildSpec ID"=w461) -> ("error out"=w462:errorcluster)  [unwired: 2 in, 4 out]
                n178 = call <vilib>:"MPU_ASWServer_Send.vi"("generate events? (F)"=TRUE, "wait for ACK (T)"=FALSE, "buildSpec ID"=w461, "error in"=w462, "control value"=path "", "control name"="path to map file", "tab name"="Build Report") -> ()  [unwired: 5 out]
              }
              frame 27 {
                w515 = "Output" ("tab name")
                n179 = Get Date/Time In Seconds() -> (seconds since 1Jan1904=w509:timestamp)
                n180 = Get Date/Time String(seconds (now)=w509, want seconds? (F)=TRUE) -> (time string=w513:string)  [unwired: 2 out]
                n181 = Concatenate Strings("[" ("string"), w513, "]" ("string"), " Status: Build Cancelled." ("string"), "\r\n") -> (w518:string)
                n182 = call <vilib>:"MPU_ASWServer_Send.vi"("generate events? (F)"=TRUE ("show tab? (F)"), "wait for ACK (T)"=FALSE, "buildSpec ID"=w500, "error in"=w507, "control value"=w518, "control name"=w515, "tab name"=w515) -> ("error out"=w506:errorcluster)  [unwired: 4 out]
                n183 = call-poly <vilib>:"MPU_ASWServer_General_SetProgressBar.vi"("buildSpec ID"=w500, "error in"=w506, "title"="Cancelled") -> ("error out"=w520:errorcluster)  [unwired: 6 in, 2 out]
                n184 = call <vilib>:"MPU_ASWServer_General_SetCtrl.vi"("buildSpec ID"=w500, "error in"=w520, "icon"=MPU_ASWServer_GeneralIcons."Stopped" ("Icon"), "value"="Build Cancelled" ("Value"), "control"=MPU_ASWServer_GeneralCtrls."Build Status" ("Control")) -> ("error out"=w503:errorcluster)  [unwired: 4 in, 2 out]
                n185 = call <vilib>:"MPU_ASWServer_Send.vi"("generate events? (F)"=TRUE, "wait for ACK (T)"=FALSE, "buildSpec ID"=w500, "error in"=w503, "control value"=path "", "control name"="path to map file", "tab name"="Build Report") -> ()  [unwired: 5 out]
              }
            }
          }
          frame Error {
          }
        }
      }
      frame "Error", Default {
        n186 = case shown="\"NoErr\", Default" w540 {
          tunnel: ["An unexpected error occurred.\n" "A compiler error occurred.\n" "Failed to script µVision build tools." "Error generating debug information."] -> w538
          frame "NoErr", Default {
          }
          frame "CompileErr" {
          }
          frame "BildToolsErr" {
          }
          frame "DebugInfoErr" {
          }
        }
        n187 = Unbundle By Name(w539) -> ("source"=w545:string, "code"=w544:i32)
        n188 = global read "LEP_RV_LaunchGlobals.vi" "buildSpec ID"() -> (w528:string)
        n189 = Number To Decimal String(number=w544) -> (decimal integer string=w535:string)  [unwired: 1 out]
        n190 = call <vilib>:"MPU_ASWServer_General_SetCtrl.vi"("buildSpec ID"=w528, "icon"=MPU_ASWServer_GeneralIcons."Error", "value"="Build Failed", "control"=MPU_ASWServer_GeneralCtrls."Build Status") -> ("error out"=w532:errorcluster)  [unwired: 5 in, 2 out]
        n191 = Concatenate Strings(w538, w545, "\r\n", " (" ("string"), w535, ")" ("string")) -> (w533:string)
        n192 = call <vilib>:"MPU_ASWServer_Output_SetError.vi"("error in"=w532, "error str"=w533, "buildSpec ID"=w528) -> ()  [unwired: 2 in, 5 out]
      }
    }
    n193 = Equal?(x=T3."NoErr" ("Errors"), y=w24) -> (x = y?=w30:bool)
    n194 = Select(t=w29, s=w30, f=T4."Error" ("Phase")) -> (s? t:f=w27:T4)
    n195 = Equal?(x=w27, y=T4."Done" ("Phase")) -> (x = y?=w28:bool)
  }
  "error out" <- w12
  "Build Result" <- w2
  n196 = call <vilib>:"Application Directory.vi"() -> ("Application Directory"=w7:path)
  n197 = Build Path(base path=w7, name or relative path="XML_Generator_For_Performance_Measuring") -> (appended path=w5:path)
  n198 = call <vilib>:"Check if File or Folder Exists.vi"("path"=w5) -> ("error out"=w3:errorcluster, "file or folder exists?"=w4:bool)  [unwired: 8 in, 1 out]
  n199 = case "If want to make performance measurements \nGenerate XML file from linker map file" shown="True" w4 {
    tunnel: w5 -> [_ w552]
    tunnel: w2 -> [_ w553]
    tunnel: w3 -> [_ w551]
    tunnel: [_ w550] -> w1
    frame False {
    }
    frame True {
      n200 = case shown="\"Build Successful\", Default" w553 {
        tunnel: w552 -> [w561 _]
        tunnel: w551 -> [w557 _]
        tunnel: [w554 _] -> w550
        frame "Build Successful", Default {
          n201 = Build Path(base path=w561, name or relative path="LEP_RV_GenerateXMLFromLinkerMapFile.vi") -> (appended path=w566:path)
          n202 = global read "LEP_RV_LaunchGlobals.vi" "Config"() -> (w559:T9)
          n203 = global read "LEP_RV_LaunchGlobals.vi" "UV Project File"() -> (w558:path)
          n204 = Unbundle By Name(w559) -> ("Compiler Flags"=w556:string)
          n205 = Unbundle By Name(w559) -> ("Linker Flags"=w555:string)
          n206 = Open VI Reference(type specifier VI Refnum (for type only)=refnum<vi> refnum ("Growable Node with Header"), vi path=w566, error in (no error)=w557) -> (vi reference=w562:refnum<vi>, error out=w563:errorcluster)  [unwired: 3 in]
          n207 = call-by-ref "?"(reference=w562, error in=w563, "Linker flags"=w555, "Compiler flags"=w556, "Project path"=w558) -> (reference out=w565:refnum<vi>, error out=w564:errorcluster)  [unwired: 9 in]
          n208 = Close Reference(reference=w565, error in (no error)=w564) -> (error out=w554:errorcluster)
        }
        frame "Build Failed" {
        }
      }
    }
  }
  n209 = call <vilib>:"Clear Errors.vi"("error in (no error)"=w1) -> ("error out"=w8:errorcluster)  [unwired: 6 in]
  n210 = global read "LEP_RV_LaunchGlobals.vi" "buildSpec ID"() -> (w9:string)
  n211 = call <vilib>:"MPU_ASWServer_SetBusy.vi"("buildSpec ID"=w9, "error in (no error)"=w8, "message"=MPU_ASWServer_Messages."NoMessage", "action"=enum32{"Clear", "Set"}."Clear") -> ()  [unwired: 6 out]
